vi "GSP_Manager_F1.vi"() -> ()   [LabVIEW 2015]
uses:
  SystemUtil/Command.ctl
  SystemUtil/ScriptArray.ctl
  SystemUtil/Script.ctl
  SystemUtil/MotorStates.ctl
  SystemUtil/ThreadStates.ctl
  Log/LogItem.ctl
  GSP_F1_Global.vi
  GUI/GSP_GUI_global.vi
panel:
  out "5-hole wheel instead of 6?":bool
  in  "Primary Filter":i32(ring) items=["<NO FILTER>", "W012", "g-SDSS", "r-SDSS", "i-SDSS"]
  out "Last Error":errorcluster
  in  "CommandQ":string
  # "Primary Filter"
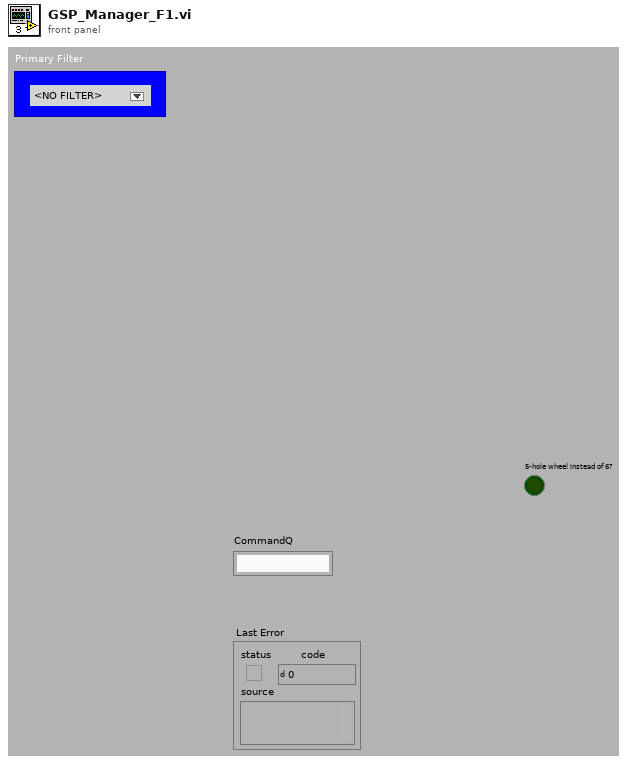
[diagram p1: front panel]
types:
  T1 = typedef "Command.ctl" = cluster{"Command":string, "Parameter":string}
  T2 = typedef "ScriptArray.ctl" = T3[]
  T3 = typedef "Script.ctl" = cluster{"Current Step":i32, "Commands":cluster{"Command":string, "Parameters":string}[]}
  T4 = cluster{"Move Mem Address":i32, "Home Mem Address":i32}
  T5 = typedef "MotorStates.ctl" = enum16{"Ready", "Moving", "Uninitialized", "Error"}
  T6 = typedef "ThreadStates.ctl" = enum16{"Waiting", "Scripting", "Uninitialized", "Error"}
  T7 = typedef "LogItem.ctl" = cluster{"error in (no error)":errorcluster, "Source":string, "Comment ":string}
  T8 = enum16{"Launch", "Log", "Open", "Close", "Shutdown"}
  T9 = enum16{"POL (0)", "CPL (1)", "HLT (2)", "STP (3)", "RST (4)", "RVN (5)", "RPB (6)", "CLP (8)", "SDL (9)", "RUN (10)", "WRI (11)", "RRG (12)", "SPR (13)", "LPR (14)", "VMI (15)", "SSP (17)", "SSE (18)", "RIS (20)", "RIO (21)", "IMW (25)", "END (128)", "MAV (134)", "MRV (135)", "JRE (137)", "WCL (138)", "WCW (139)", "DLY (140)", "WDL (141)", "GCL (142)", "GOP (143)", "ZTG (144)", "ZTP (145)", "TTP (146)", "CME (147)", "CTC (148)", "TQL (149)", "AHC (150)", "ERL (151)", "OLP (152)", "WRP (154)", "IDT (155)", "LRP (156)", "VMP (159)", "RAV (160)", "RRV (161)", "JMP (162)", "JOI (162)", "CIS (163)", "CKS (164)", "CLC (165)", "KMC (167)", "MCT (168)", "FLC (169)", "EEM (170)", "DDB (171)", "DEM (171)", "PAC (172)", "ADL (173)", "BRT (174)", "MAT (176)", "MRT (177)", "RAT (178)", "RRT (179)", "SSD (180)", "KMR (181)", "KED (182)", "KDD (183)", "DIR (184)", "PRO (185)", "SIF (186)", "EDL (187)", "CIO (188)", "MDS (189)", "MDC (190)", "MDT (191)", "SEE (192)", "ARI (193)", "WBS (194)", "SCF (195)", "RSM (196)", "RLM (197)", "RSN (198)", "RLN (199)", "PCL (201)", "PCI (201)", "PRT (202)", "PRI (202)", "WBE (204)", "SOB (205)", "COB (206)", "ACR (207)", "PLR (208)", "CAI (211)", "LVT (212)", "OVT (213)", "MTT (214)", "CLC (215)", "PIM (216)", "VIM (217)", "TIM (218)", "AHM (219)", "SSL (221)", "TRU (222)", "RSD (223)", "EMT (225)", "DMT (226)", "EMD (227)", "DMD (228)", "HSM (229)", "AHD (230)", "PCM (231)", "PCG (232)", "XRV (233)", "XAV (234)", "XRT (235)", "XAT (236)", "GOC (237)", "JNA (238)", "JOR (239)", "PMC (240)", "PMV (241)", "PMX (242)", "DLC (243)", "SLC (244)", "PCP (245)", "ATR (248)", "PMO (249)", "JAN (250)", "EDH (251)", "DIF (252)", "IMS (253)", "IMQ (254)"}
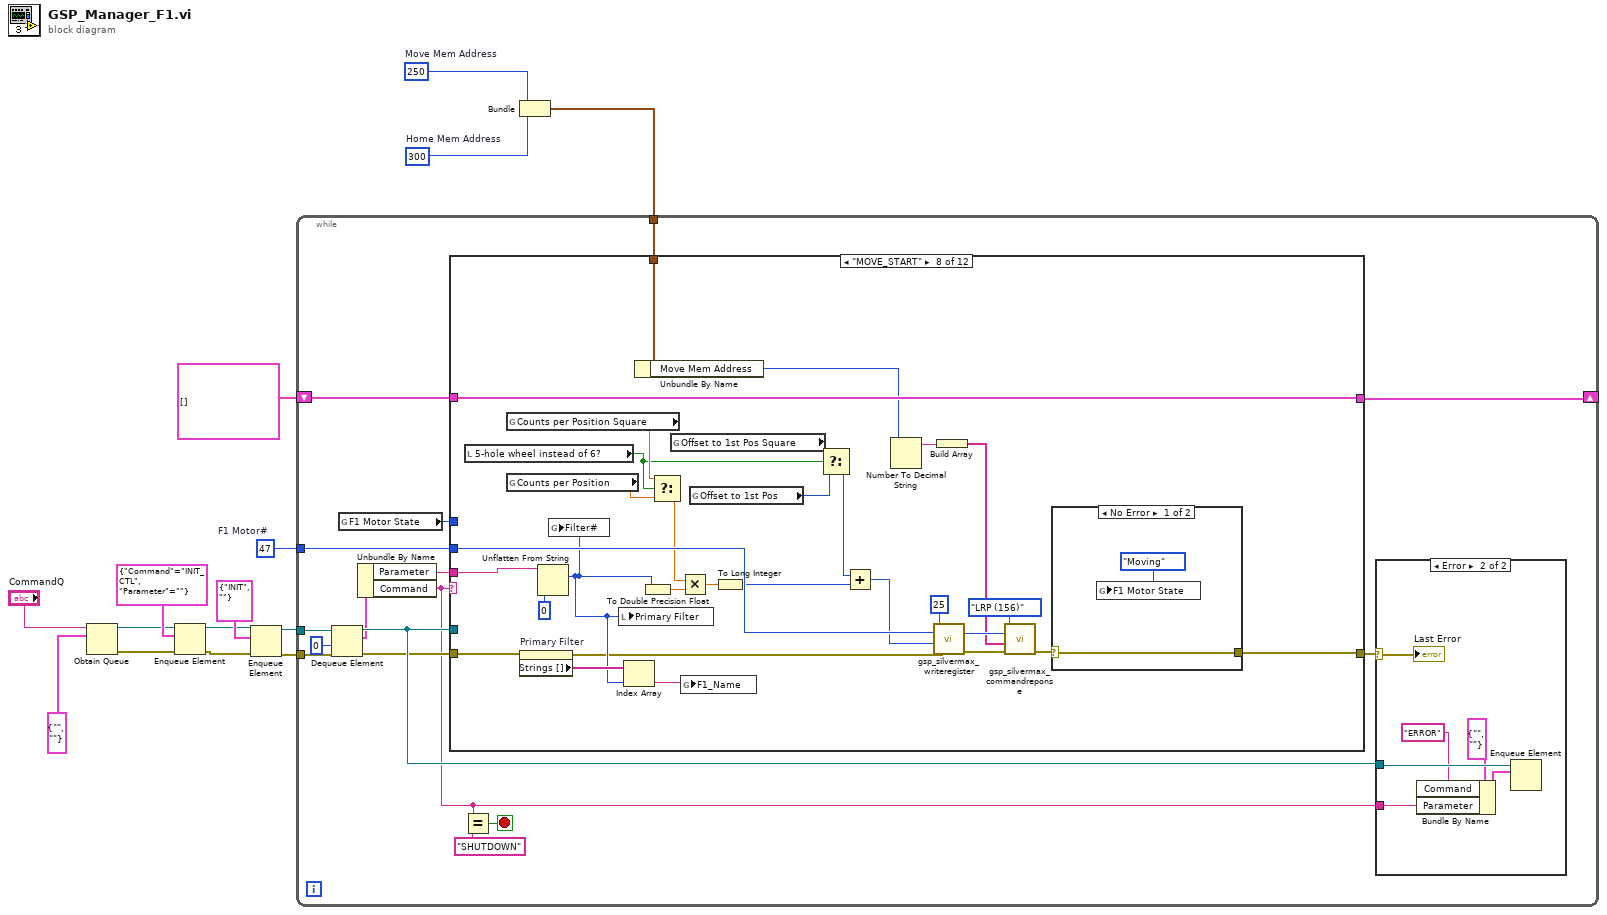
[diagram p0: block diagram]
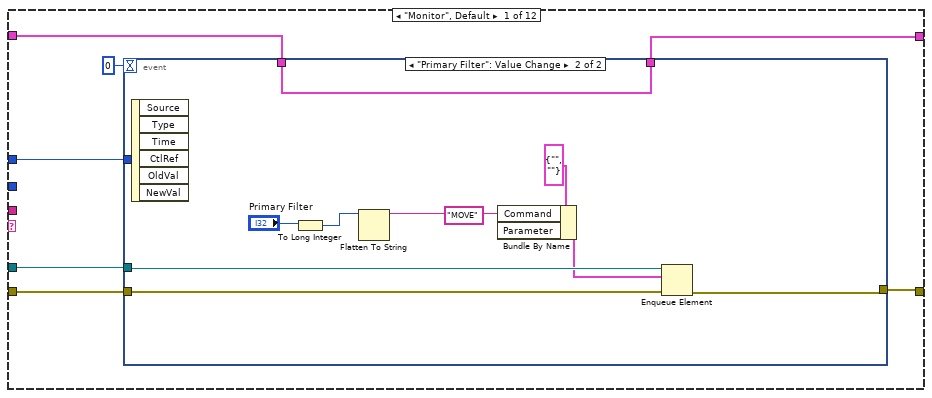
[diagram p3: hidden frame]
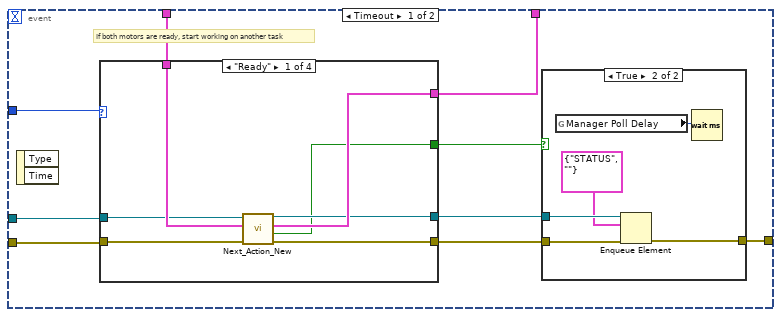
[diagram p4: hidden frame]
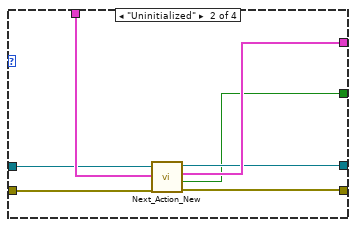
[diagram p6: hidden frame]
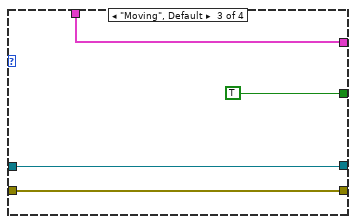
[diagram p7: hidden frame]
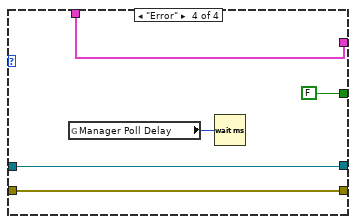
[diagram p8: hidden frame]
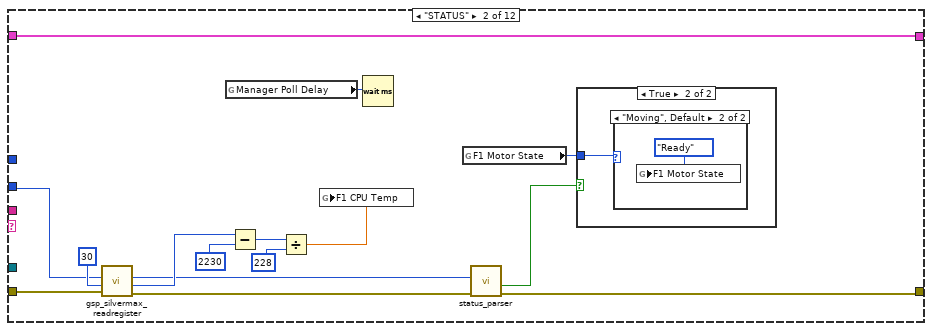
[diagram p9: hidden frame]
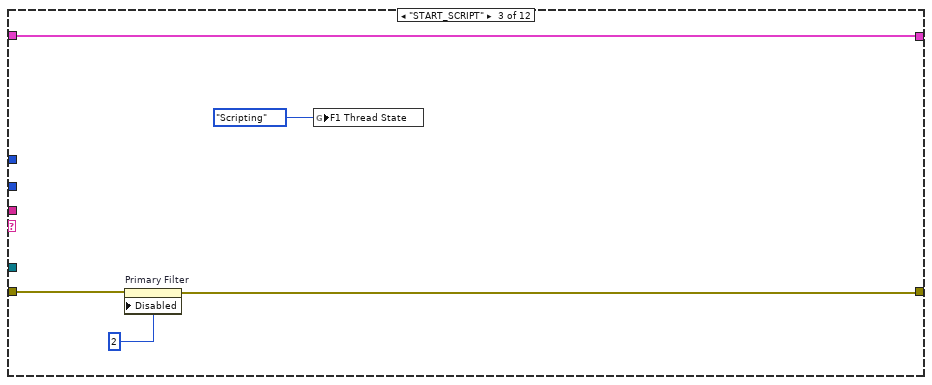
[diagram p12: hidden frame]
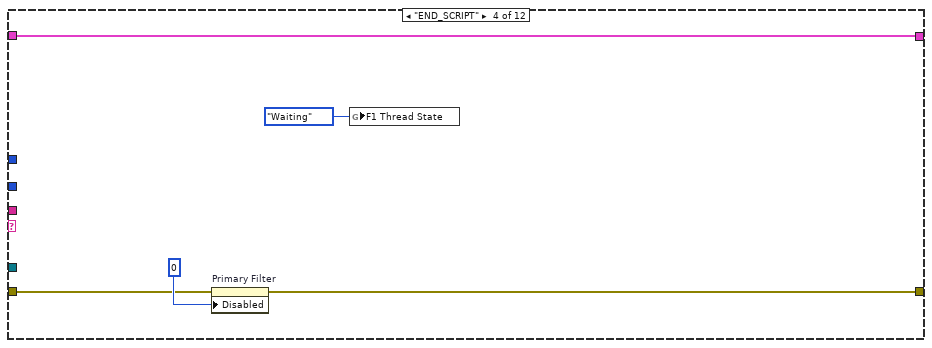
[diagram p13: hidden frame]
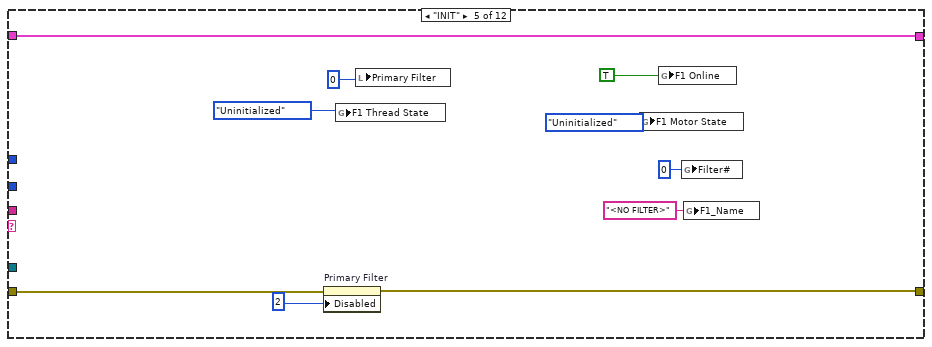
[diagram p14: hidden frame]
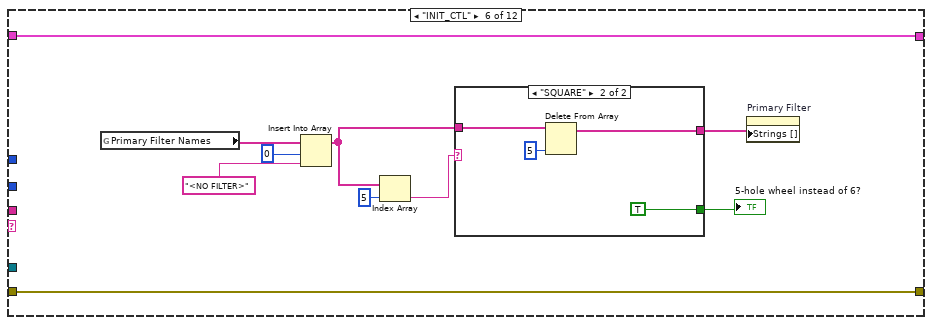
[diagram p15: hidden frame]
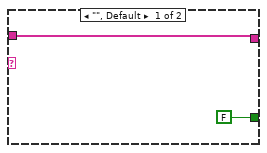
[diagram p16: hidden frame]
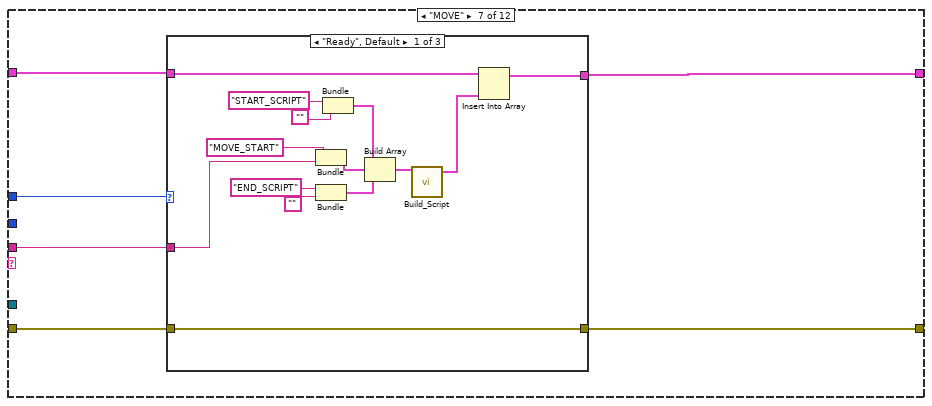
[diagram p17: hidden frame]
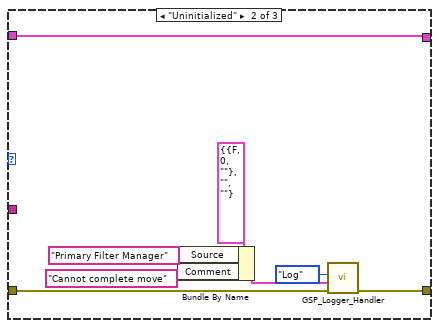
[diagram p18: hidden frame]
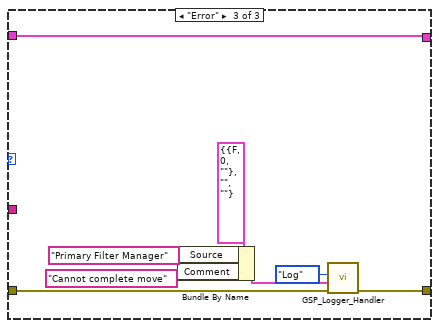
[diagram p19: hidden frame]
diagram:
  w9 = 300  # Home Mem Address
  w10 = 250  # Move Mem Address
  w14 = u8 47  # F1 Motor#
  n1 = Obtain Queue(name (unnamed)="CommandQ", element data type=T1 {"Command"="", "Parameter"=""} ("Command")) -> (queue out=w2:refnum<queue>, error out=w1:errorcluster)  [unwired: 3 in, 1 out]
  n2 = Enqueue Element(queue=w2, element=T1 {"Command"="INIT_CTL", "Parameter"=""}, error in (no error)=w1) -> (queue out=w4:refnum<queue>, error out=w3:errorcluster)  [unwired: 1 in, 1 out]
  n3 = Enqueue Element(queue=w4, element=T1 {"Command"="INIT", "Parameter"=""}, error in (no error)=w3) -> (queue out=w7:refnum<queue>, error out=w6:errorcluster)  [unwired: 1 in, 1 out]
  n4 = Bundle("Move Mem Address"=w10, "Home Mem Address"=w9) -> (w8:T4)  [unwired: 1 in]
  n5 = while {
    tunnel: w7 -> [w31]
    tunnel: w6 -> [w30]
    tunnel: w14 -> [w25]
    shift-right: [w23] -> _
    shift-left: T2 [] ("Operations") -> [w24]
    tunnel: w8 -> [w16]
    stop <- w19 stop-if-true
    n6 = Dequeue Element(queue=w31, timeout in ms (-1)=0, error in (no error)=w30) -> (queue out=w28:refnum<queue>, element=w21:T1, error out=w26:errorcluster)  [unwired: 1 out]
    n7 = global read "GSP_F1_Global.vi" "F1 Motor State"() -> (w17:T5)
    n8 = Unbundle By Name(w21) -> ("Parameter"=w20:string, "Command"=w18:string)
    n9 = case shown="\"MOVE_START\"" w18 {
      tunnel: w26 -> [w43 w97 w113 w117 w125 w135 w149 w193 w220 w242 w245 _]
      tunnel: w28 -> [w44 _ _ _ _ _ _ _ w219 _ _ w266]
      tunnel: [w39 w106 w111 w116 w123 w135 w148 w203 w217 w242 w251 _] -> w29
      tunnel: w25 -> [_ w95 _ _ _ _ _ w206 _ _ w253 _]
      tunnel: w24 -> [w42 w105 w114 w119 w128 w136 w151 w200 w221 w241 w248 w259]
      tunnel: [w41 w105 w114 w119 w128 w136 w150 w200 w221 w240 w248 w258] -> w23
      tunnel: w20 -> [_ _ _ _ _ _ w147 w199 _ _ _ _]
      tunnel: w17 -> [w40 _ _ _ _ _ w146 _ _ _ _ _]
      tunnel: w16 -> [_ _ _ _ _ _ _ w195 _ _ w247 _]
      frame "Monitor", Default {
        n10 = event shown="[1] \"Primary Filter\": Value Change" {
          selector: _ -> [_ _]
          dyn-events: _ -> [_ _]
          timeout: 0 -> [_ _]
          tunnel: w44 -> [w53 w88]
          tunnel: w43 -> [w52 w89]
          tunnel: w42 -> [w51 w92]
          tunnel: [w50 w92] -> w41
          tunnel: w40 -> [w49 _]
          tunnel: [w45 w83] -> w39
          event Timeout {
            # "If both motors are ready, start working on another task"
            n11 = event-data() -> ()  [unwired: 1 in, 2 out]
            n12 = case shown="\"Ready\"" w49 {
              tunnel: w53 -> [w62 w69 w76 w79]
              tunnel: w52 -> [w66 w73 w75 w81]
              tunnel: [w63 w70 w75 w81] -> w48
              tunnel: w51 -> [w65 w72 w77 w82]
              tunnel: [w64 w71 w77 w82] -> w50
              tunnel: [w61 w68 w76 w79] -> w47
              tunnel: [w60 w67 TRUE FALSE] -> w46
              frame "Ready" {
                n13 = call "Next_Action_New.vi"("error in (no error)"=w66, "Operations"=w65, "queue in"=w62) -> ("error out"=w63:errorcluster, "No command?"=w60:bool, "Operations Out"=w64:T2, "queue out"=w61:refnum<queue>)  [unwired: 1 in]
              }
              frame "Uninitialized" {
                n14 = call "Next_Action_New.vi"("error in (no error)"=w73, "Operations"=w72, "queue in"=w69) -> ("error out"=w70:errorcluster, "No command?"=w67:bool, "Operations Out"=w71:T2, "queue out"=w68:refnum<queue>)  [unwired: 1 in]
              }
              frame "Moving", Default {
              }
              frame "Error" {
                n15 = global read "GSP_GUI_global.vi" "Manager Poll Delay"() -> (w80:u32)
                n16 = Wait (ms)(milliseconds to wait=w80) -> ()  [unwired: 1 out]
              }
            }
            n17 = case shown="True" w46 {
              tunnel: w48 -> [w54 w59]
              tunnel: w47 -> [_ w58]
              tunnel: [w54 w57] -> w45
              frame False {
              }
              frame True {
                n18 = global read "GSP_GUI_global.vi" "Manager Poll Delay"() -> (w56:u32)
                n19 = Enqueue Element(queue=w58, element=T1 {"Command"="STATUS", "Parameter"=""}, error in (no error)=w59) -> (error out=w57:errorcluster)  [unwired: 1 in, 2 out]
                n20 = Wait (ms)(milliseconds to wait=w56) -> ()  [unwired: 1 out]
              }
            }
          }
          event "Primary Filter": Value Change {
            n21 = event-data() -> ()  [unwired: 1 in, 6 out]
            n22 = To Long Integer(number="Primary Filter") -> (32bit integer=w84:i32)
            n23 = Flatten To String(anything=w84) -> (data string=w90:string)  [unwired: 3 in, 2 out]
            n24 = Bundle By Name(cluster=T1 {"Command"="", "Parameter"=""} ("element"), "Command"="MOVE" ("element"), "Parameter"=w90) -> (w86:T1)
            n25 = Enqueue Element(queue=w88, element=w86, error in (no error)=w89) -> (error out=w83:errorcluster)  [unwired: 1 in, 2 out]
          }
        }
      }
      frame "STATUS" {
        n26 = call "gsp_silvermax_readregister.vi"("error in (no error)"=w97, "Register# (0)"=u8 30, "Motor #"=w95) -> ("error out"=w96:errorcluster, "Register Value"=w102:i32, "Motor # dup"=w94:u8)  [unwired: 2 in, 2 out]
        n27 = global read "GSP_GUI_global.vi" "Manager Poll Delay"() -> (w104:u32)
        n28 = Subtract(x=w102, y=2230) -> (x-y=w101:i32)
        n29 = Divide(x=w101, y=228) -> (x/y=w98:dbl)
        n30 = global write "GSP_F1_Global.vi" "F1 CPU Temp"(w98) -> ()
        n31 = Wait (ms)(milliseconds to wait=w104) -> ()  [unwired: 1 out]
        n32 = global read "GSP_F1_Global.vi" "F1 Motor State"() -> (w93:T5)
        n33 = call "status_parser.vi"("error in (no error)"=w96, "Motor #"=w94) -> ("error out"=w106:errorcluster, "Program Complete?"=w107:bool)  [unwired: 3 in, 1 out]
        n34 = case shown="True" w107 {
          tunnel: w93 -> [_ w108]
          frame False {
          }
          frame True {
            n35 = case shown="\"Moving\", Default" w108 {
              frame "Uninitialized" {
              }
              frame "Moving", Default {
                n36 = global write "GSP_F1_Global.vi" "F1 Motor State"(MotorStates."Ready" ("Mode")) -> ()
              }
            }
          }
        }
      }
      frame "START_SCRIPT" {
        n37 = property on="Primary Filter" class="Ring (strict)"(error in=w113, "Disabled"=u8 2) -> (error out=w111:errorcluster)  [unwired: 1 in, 1 out]
        n38 = global write "GSP_F1_Global.vi" "F1 Thread State"(ThreadStates."Scripting" ("Thread state")) -> ()
      }
      frame "END_SCRIPT" {
        n39 = property on="Primary Filter" class="Ring (strict)"(error in=w117, "Disabled"=u8 0) -> (error out=w116:errorcluster)  [unwired: 1 in, 1 out]
        n40 = global write "GSP_F1_Global.vi" "F1 Thread State"(ThreadStates."Waiting" ("Thread state")) -> ()
      }
      frame "INIT" {
        n41 = property on="Primary Filter" class="Ring (strict)"(error in=w125, "Disabled"=u8 2) -> (error out=w123:errorcluster)  [unwired: 1 in, 1 out]
        n42 = global write "GSP_F1_Global.vi" "F1 Thread State"(ThreadStates."Uninitialized" ("Thread state")) -> ()
        n43 = local write "Primary Filter"(0 ("Value")) -> ()
        n44 = global write "GSP_F1_Global.vi" "F1 Motor State"(MotorStates."Uninitialized" ("Mode")) -> ()
        n45 = global write "GSP_F1_Global.vi" "F1 Online"(TRUE ("CS Online")) -> ()
        n46 = global write "GSP_F1_Global.vi" "Filter#"(0 ("Filter Position")) -> ()
        n47 = global write "GSP_F1_Global.vi" "F1_Name"("<NO FILTER>" ("F1_Name")) -> ()
      }
      frame "INIT_CTL" {
        n48 = global read "GSP_GUI_global.vi" "Primary Filter Names"() -> (w138:string[])
        n49 = Insert Into Array(array=w138, index=0, new element="<NO FILTER>" ("new element/subarray")) -> (w134:string[])
        n50 = Index Array(array=w134, index=5) -> (element=w132:string)
        n51 = case shown="\"SQUARE\"" w132 {
          tunnel: w134 -> [w141 w145]
          tunnel: [w141 w143] -> w131
          tunnel: [FALSE ("5 hole or 6 hole wheel?") TRUE ("5 hole or 6 hole wheel?")] -> w130
          frame "", Default {
          }
          frame "SQUARE" {
            n52 = Delete From Array(array=w145, index=5) -> (array with subset deleted=w143:string[])  [unwired: 1 in, 1 out]
          }
        }
        "5-hole wheel instead of 6?" <- w130
        n53 = property on="Primary Filter" class="Ring (strict)"("Strings []"=w131) -> ()  [unwired: 2 in, 2 out]
      }
      frame "MOVE" {
        n54 = case shown="\"Ready\", Default" w146 {
          tunnel: w151 -> [w165 w173 w181]
          tunnel: [w164 w173 w181] -> w150
          tunnel: w149 -> [w163 w172 w180]
          tunnel: [w163 w171 w179] -> w148
          tunnel: w147 -> [w157 _ _]
          frame "Ready", Default {
            n55 = Bundle("MOVE_START", "Parameter"=w157) -> (w156:cluster{string, "Parameter":string})  [unwired: 1 in]
            n56 = Bundle("END_SCRIPT", "") -> (w159:cluster{string, string})  [unwired: 1 in]
            n57 = Bundle("START_SCRIPT", "") -> (w152:cluster{string, string})  [unwired: 1 in]
            n58 = Build Array(w152, w156, w159) -> (w158:cluster{string, "Parameter":string}[])
            n59 = call "Build_Script.vi"("Commands"=w158) -> ("script out"=w155:T3)  [unwired: 4 in]
            n60 = Insert Into Array(array=w165, new element=w155) -> (w164:T2)  [unwired: 1 in]
          }
          frame "Uninitialized" {
            n61 = Bundle By Name(cluster=T7 {"error in (no error)"={"status"=FALSE, "code"=0, "source"=""}, "Source"="", "Comment "=""} ("Log"), "Source"="Primary Filter Manager", "Comment"="Cannot complete move") -> (w168:T7)
            n62 = call "GSP_Logger_Handler.vi"("error in (no error)"=w172, "Log"=w168, "Actions"=T8."Log") -> ("error out"=w171:errorcluster)  [unwired: 4 in]
          }
          frame "Error" {
            n63 = Bundle By Name(cluster=T7 {"error in (no error)"={"status"=FALSE, "code"=0, "source"=""}, "Source"="", "Comment "=""} ("Log"), "Source"="Primary Filter Manager", "Comment"="Cannot complete move") -> (w176:T7)
            n64 = call "GSP_Logger_Handler.vi"("error in (no error)"=w180, "Log"=w176, "Actions"=T8."Log") -> ("error out"=w179:errorcluster)  [unwired: 4 in]
          }
        }
      }
      frame "MOVE_START" {
        n65 = local read "5-hole wheel instead of 6?"() -> (w186:bool)
        n66 = global read "GSP_F1_Global.vi" "Counts per Position Square"() -> (w187:dbl)
        n67 = global read "GSP_F1_Global.vi" "Counts per Position"() -> (w188:dbl)
        n68 = property on="Primary Filter" class="Ring (strict)"(error in=w193) -> (error out=w190:errorcluster, "Strings []"=w192:string[])  [unwired: 1 in, 1 out]
        n69 = Unflatten From String(type=0, binary string=w199) -> (value=w191:i32)  [unwired: 3 in, 2 out]
        n70 = global write "GSP_F1_Global.vi" "Filter#"(w191) -> ()
        n71 = local write "Primary Filter"(w191) -> ()
        n72 = Index Array(array=w192, index=w191) -> (element=w189:string)
        n73 = Unbundle By Name(w195) -> ("Move Mem Address"=w194:i32)
        n74 = To Double Precision Float(number=w191) -> (double precision float=w211:dbl)
        n75 = Select(t=w187, s=w186, f=w188) -> (s? t:f=w182:dbl)
        n76 = global read "GSP_F1_Global.vi" "Offset to 1st Pos Square"() -> (w184:i32)
        n77 = Multiply(x=w182, y=w211) -> (x*y=w210:dbl)
        n78 = global write "GSP_F1_Global.vi" "F1_Name"(w189) -> ()
        n79 = global read "GSP_F1_Global.vi" "Offset to 1st Pos"() -> (w185:i32)
        n80 = To Long Integer(number=w210) -> (32bit integer=w197:i32)
        n81 = Select(t=w184, s=w186, f=w185) -> (s? t:f=w183:i32)
        n82 = Add(x=w183, y=w197) -> (x+y=w196:i32)
        n83 = Number To Decimal String(number=w194) -> (decimal integer string=w202:string)  [unwired: 1 in]
        n84 = call "gsp_silvermax_writeregister.vi"("error in (no error)"=w190, "Register Value"=w196, "Motor #"=w206, "Register# (0)"=u8 25) -> ("error out"=w208:errorcluster, "Motor # dup"=w207:u8)  [unwired: 2 in]
        n85 = Build Array(w202) -> (w201:string[])
        n86 = call "gsp_silvermax_commandreponse.vi"("error in (no error)"=w208, "Parameters (none)"=w201, "Motor #"=w207, "Command"=T9."LRP (156)") -> ("error out"=w204:errorcluster)  [unwired: 3 out]
        n87 = case shown="No Error" w204 {
          selector: w204 -> [w213 w214]
          tunnel: [w213 w214] -> w203
          frame No Error {
            n88 = global write "GSP_F1_Global.vi" "F1 Motor State"(MotorStates."Moving" ("Mode")) -> ()
          }
          frame Error {
          }
        }
      }
      frame "SHUTDOWN" {
        n89 = Release Queue(queue=w219, error in (no error)=w220) -> (error out=w215:errorcluster)  [unwired: 1 in, 2 out]
        n90 = global write "GSP_F1_Global.vi" "F1 Thread State"(ThreadStates."Uninitialized" ("Thread state")) -> ()
        n91 = property on="Primary Filter" class="Ring (strict)"(error in=w215, "Disabled"=u8 2) -> (error out=w217:errorcluster)  [unwired: 1 in, 1 out]
        n92 = stacked-sequence {
          frame #0 {
            n93 = global write "GSP_F1_Global.vi" "F1 Online"(FALSE ("CS Online")) -> ()
          }
        }
      }
      frame "HOME" {
        n94 = To Long Integer(number=0) -> (32bit integer=w225:i32)
        n95 = Flatten To String(anything=w225) -> (data string=w227:string)  [unwired: 3 in, 2 out]
        n96 = Bundle("START_SCRIPT", "") -> (w229:cluster{string, string})  [unwired: 1 in]
        n97 = Bundle("HOME_START", "") -> (w235:cluster{string, string})  [unwired: 1 in]
        n98 = Bundle("END_SCRIPT", "") -> (w234:cluster{string, string})  [unwired: 1 in]
        n99 = Bundle By Name(cluster=T1 {"Command"="", "Parameter"=""} ("element"), "Command"="MOVE" ("element"), "Parameter"=w227) -> (w223:T1)
        n100 = Build Array(w229, w235, w234, w223) -> (w233:T1[])
        n101 = call "Build_Script.vi"("Commands"=w233) -> ("script out"=w232:T3)  [unwired: 4 in]
        n102 = Insert Into Array(array=w241, new element=w232) -> (w240:T2)  [unwired: 1 in]
      }
      frame "HOME_START" {
        w243 = 0 ("Value")
        n103 = Unbundle By Name(w247) -> ("Home Mem Address"=w246:i32)
        n104 = Number To Decimal String(number=w246) -> (decimal integer string=w250:string)  [unwired: 1 in]
        n105 = Build Array(w250) -> (w249:string[])
        n106 = call "gsp_silvermax_commandreponse.vi"("error in (no error)"=w245, "Parameters (none)"=w249, "Motor #"=w253, "Command"=T9."LRP (156)") -> ("error out"=w254:errorcluster)  [unwired: 3 out]
        n107 = case shown="No Error" w254 {
          selector: w254 -> [w256 w257]
          tunnel: [w256 w257] -> w251
          frame No Error {
            n108 = global write "GSP_F1_Global.vi" "F1 Motor State"(MotorStates."Moving" ("Mode")) -> ()
          }
          frame Error {
          }
        }
        n109 = local write "Primary Filter"(w243) -> ()
        n110 = global write "GSP_F1_Global.vi" "F1_Name"("<NO FILTER>" ("F1_Name")) -> ()
        n111 = global write "GSP_F1_Global.vi" "Filter#"(w243) -> ()
      }
      frame "ERROR" {
        n112 = local read "Last Error"() -> (w261:errorcluster)
        n113 = Unbundle By Name(w261) -> ("code"=w267:i32)
        n114 = Bundle By Name(cluster=T7 {"error in (no error)"={"status"=FALSE, "code"=0, "source"=""}, "Source"="", "Comment "=""} ("Log"), "error in (no error)"=w261, "Source"="Primary Filter Manager") -> (w263:T7)
        n115 = call "GSP_Logger_Handler.vi"("Log"=w263, "Actions"=T8."Log") -> ()  [unwired: 5 in, 1 out]
        n116 = case shown="5003, 5006" w267 {
          tunnel: w261 -> [_ _ _]
          tunnel: [errorcluster {"status"=FALSE, "code"=0, "source"=""} ("error IO") errorcluster {"status"=FALSE, "code"=0, "source"=""} ("error IO") errorcluster {"status"=FALSE, "code"=0, "source"=""} ("error IO")] -> w260
          tunnel: w259 -> [_ w276 w278]
          tunnel: [T2 [] ("Operations") w276 w278] -> w258
          frame 0, Default {
            n117 = global write "GSP_F1_Global.vi" "F1 Motor State"(MotorStates."Error" ("Mode")) -> ()
            n118 = property on="Primary Filter" class="Ring (strict)"("Disabled"=u8 2) -> ()  [unwired: 2 in, 2 out]
            n119 = global write "GSP_F1_Global.vi" "F1 Thread State"(ThreadStates."Error" ("Thread state")) -> ()
          }
          frame 5003, 5006 {
          }
          frame 5013 {
          }
        }
        n120 = case shown="Error" w260 {
          tunnel: w266 -> [_ w269]
          frame No Error {
          }
          frame Error {
            n121 = Enqueue Element At Opposite End(queue=w269, element=T1 {"Command"="SHUTDOWN", "Parameter"=""}) -> ()  [unwired: 2 in, 3 out]
          }
        }
      }
    }
    n122 = Equal?(x=w18, y="SHUTDOWN") -> (x = y?=w19:bool)
    n123 = case shown="Error" w29 {
      selector: w29 -> [_ w36]
      tunnel: w28 -> [_ w37]
      tunnel: w18 -> [_ w33]
      frame No Error {
      }
      frame Error {
        n124 = Bundle By Name(cluster=T1 {"Command"="", "Parameter"=""} ("element"), "Command"="ERROR" ("element"), "Parameter"=w33) -> (w35:T1)
        n125 = Enqueue Element(queue=w37, element=w35) -> ()  [unwired: 2 in, 3 out]
        "Last Error" <- w36
      }
    }
  }
